vi "Collect U256 on Datavalid.vi"(9 "Data Valid":bool, 10 "Input Data":T1) -> (2 "Collected Data":T1[](array[typedef]))   [LabVIEW 2011]
uses:
  Code Development/DRAM/2 Bank DRAM/Data Type (256).ctl
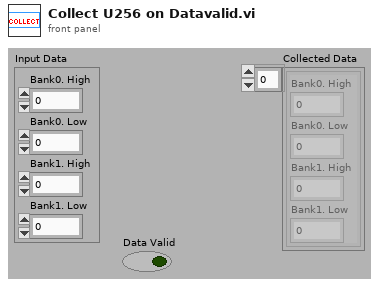
[diagram p1: front panel]
types:
  T1 = typedef "Data Type (256).ctl" = cluster{"Bank0. High":u64, "Bank0. Low":u64, "Bank1. High":u64, "Bank1. Low":u64}
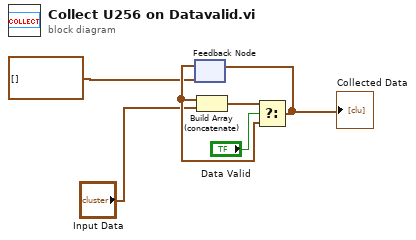
[diagram p0: block diagram]
diagram:
  n1 = feedback #1(T1[] []) -> (w5:T1[])
  n2 = Build Array (concatenate)(w5, "Input Data") -> (w6:T1[])
  n3 = Select(t=w6, s="Data Valid", f=w5) -> (s? t:f=w1:T1[])
  "Collected Data" <- w1
  n4 = feedback-in #1(w1) -> ()
